vi "Set Log Instance and ID.vi"(9 "Log Alias":string, 10 "Log Instance":refnum<class "LoggerReference.lvclass">, 11 "LoggedActor in":refnum<class "LoggedActor.lvclass">) -> (3 "LoggedActor out":refnum<class "LoggedActor.lvclass">)   [LabVIEW 2020, in "LoggedActor.lvclass"]
uses:
  <vilib>/gpm_packages/@cs/Network-interface/Source/Logged Actor/LoggedActor.lvclass
  <vilib>/gpm_packages/@cs/event-logger/Source/Composed Log/LoggerReference/LoggerReference.lvclass
  <vilib>/gpm_packages/@cs/Network-interface/Source/Logged Actor/LoggedActor.lvclass/LoggedActor.ctl
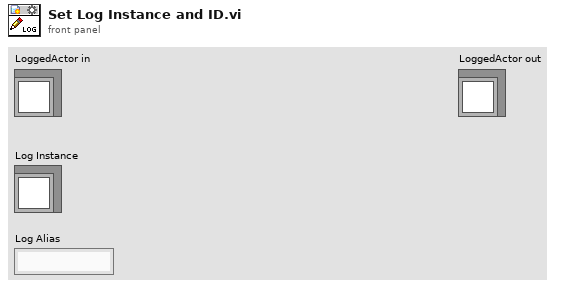
[diagram p1: front panel]
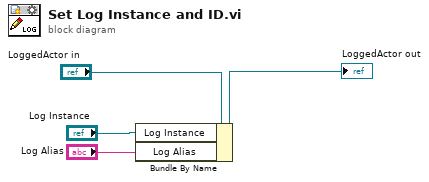
[diagram p0: block diagram]
diagram:
  n1 = Bundle By Name(cluster="LoggedActor in", "Log Instance"="Log Instance", "Log Alias"="Log Alias") -> (→"LoggedActor out":refnum<class "LoggedActor.lvclass">)
